vi "Stop OPC UA.vi"(8 "error in (no error)":errorcluster, 11 "SM EOL Station Actor in":refnum<class "PLC Sim Controller Actor.lvclass">) -> (0 "error out":errorcluster, 3 "SM EOL Station Actor out":refnum<class "PLC Sim Controller Actor.lvclass">)   [LabVIEW 2019, in "PLC Sim Controller Actor.lvlib" / "PLC Sim Controller Actor.lvclass"]
uses:
  PLC Sim Controller Actor.lvclass
  PLC Sim Controller Actor.lvclass/PLC Sim Controller Actor.ctl
  <vilib>/OPCUA/NI OPC UA Server.lvlib
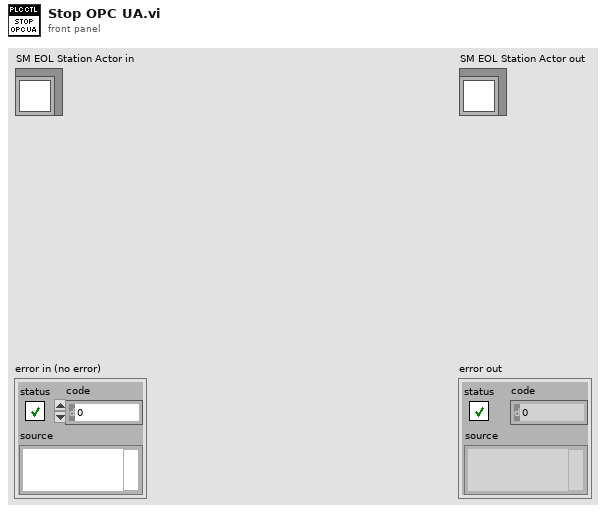
[diagram p1: front panel]
types:
  T1 = typedef "OPC UA Server Refnum.ctl" = refnum<k21>
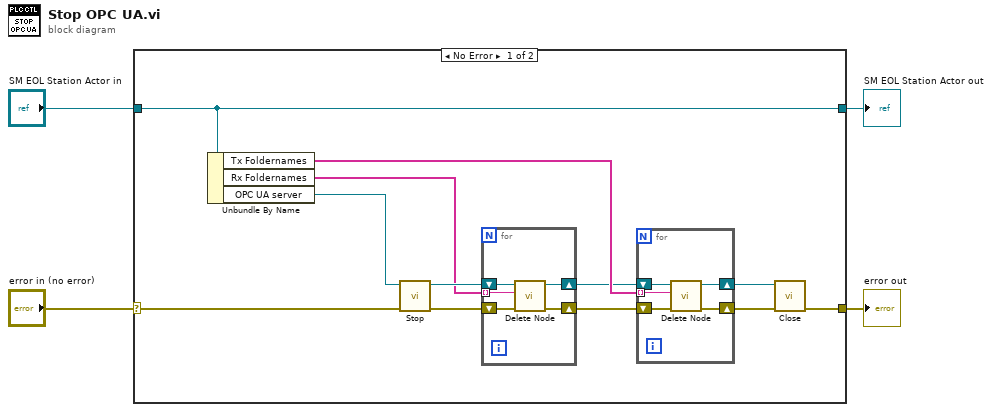
[diagram p0: block diagram]
diagram:
  n1 = case shown="No Error" "error in (no error)" {
    selector: "error in (no error)" -> [w16 w28]
    tunnel: [w6 w28] -> w3
    tunnel: [w15 w27] -> w1
    tunnel: "SM EOL Station Actor in" -> [w15 w27]
    frame No Error {
      n2 = Unbundle By Name(w15) -> ("Tx Foldernames"=w9:string[], "Rx Foldernames"=w11:string[], "OPC UA server"=w14:T1)
      n3 = call <vilib>:"Stop.vi"("error in (no error)"=w16, "OPC UA server refnum in"=w14) -> ("error out"=w13:errorcluster, "OPC UA server refnum out"=w12:T1)  [unwired: 8 in]
      n4 = for {
        tunnel: w11 -> [w24] mode=indexing
        shift-right: [w23] -> w10
        shift-left: w13 -> [w26]
        shift-right: [w22] -> w8
        shift-left: w12 -> [w25]
        n5 = call <vilib>:"Delete Node.vi"("error in (no error)"=w26, "node ID"=w24, "OPC UA server refnum in"=w25) -> ("error out"=w23:errorcluster, "OPC UA server refnum out"=w22:T1)  [unwired: 7 in]
      }
      n6 = for {
        tunnel: w9 -> [w20] mode=indexing
        shift-right: [w18] -> w7
        shift-left: w10 -> [w21]
        shift-right: [w17] -> w5
        shift-left: w8 -> [w19]
        n7 = call <vilib>:"Delete Node.vi"("error in (no error)"=w21, "node ID"=w20, "OPC UA server refnum in"=w19) -> ("error out"=w18:errorcluster, "OPC UA server refnum out"=w17:T1)  [unwired: 7 in]
      }
      n8 = call <vilib>:"Close.vi"("error in (no error)"=w7, "OPC UA server refnum in"=w5) -> ("error out"=w6:errorcluster)  [unwired: 9 in]
    }
    frame Error {
    }
  }
  "error out" <- w3
  "SM EOL Station Actor out" <- w1
